vi "Generate User Event.vi"(6 "priority (normal)":T1, 8 "error in":errorcluster, 10 "IMessagePayload.lvclass":refnum<class "IMessagePayload.lvclass">, 11 "UserEventMessageTransport":refnum<class "UserEventMessageTransport.lvclass">) -> (0 "error out":errorcluster, 3 "UserEventMessageTransport":refnum<class "UserEventMessageTransport.lvclass">)   [LabVIEW 2016, in "UserEventMessageTransport.lvclass"]
uses:
  UserEventMessageTransport.lvclass
  <vilib>/event_ctls.llb/usereventprio.ctl
  IMessagePayload/IMessagePayload.lvclass
  UserEventMessageTransport.lvclass/UserEventMessageTransport.ctl
panel:
  # "INPUTS"
  # "OUTPUTS"
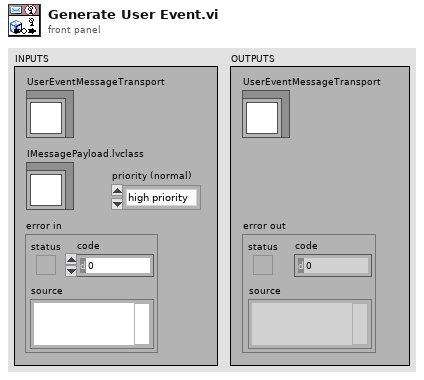
[diagram p1: front panel]
types:
  T1 = typedef "usereventprio.ctl" = enum32{"high priority", "normal priority"}
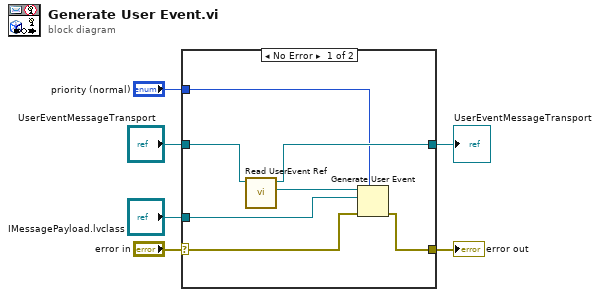
[diagram p0: block diagram]
diagram:
  n1 = case shown="No Error" "error in" {
    selector: "error in" -> [w9 w15]
    tunnel: [w7 w15] -> w5
    tunnel: [w12 w14] -> w3
    tunnel: "UserEventMessageTransport" -> [w13 w14]
    tunnel: "IMessagePayload.lvclass" -> [w10 _]
    tunnel: "priority (normal)" -> [w8 _]
    frame No Error {
      n2 = call "Read UserEvent Ref.vi"("UserEventMessageTransport in"=w13) -> ("UserEvent Ref"=w11:refnum<user-event>, "UserEventMessageTransport out"=w12:refnum<class "UserEventMessageTransport.lvclass">)  [unwired: 8 in, 1 out]
      n3 = Generate User Event(priority (normal)=w8, user event=w11, event data cluster=w10, error in=w9) -> (error out=w7:errorcluster)  [unwired: 1 out]
    }
    frame Error {
    }
  }
  "error out" <- w5
  "UserEventMessageTransport" <- w3
